vi "Read Encoder.vi"(10 "Manual Reset":bool, 11 "Encoder Ref In":T1) -> (0 "error out":errorcluster, 1 "Has Index Pulse Occured \nthis Run?":bool, 2 "Angular Encoder Abs.\nDisplacement (rad)":dbl)   [LabVIEW 2018]
uses:
  <vilib>/myRIO/Common/Instrument Driver Framework/myRIO v1.0/Encoder/typedefs/Encoder Count Direction Enum.ctl
  <vilib>/myRIO/Instrument Drivers/Onboard IO/Encoder/typedefs/Encoder Reference.ctl
  <vilib>/myRIO/Common/Instrument Driver Framework/Utilities/typedefs/myRIO Generic Hardware Reference.ctl
  <vilib>/myRIO/Common/Instrument Driver Framework/Utilities/typedefs/Hardware Version Enum.ctl
  <vilib>/myRIO/Common/Instrument Driver Framework/Utilities/typedefs/myRIO v1.0 Reference.ctl
  <vilib>/myRIO/Common/Instrument Driver Framework/Utilities/typedefs/Generic FPGA Reference.ctl
  <vilib>/myRIO/Common/Instrument Driver Framework/myRIO v1.0/Encoder/typedefs/Encoder Channels Enum.ctl
  <vilib>/Utility/error.llb/Error Cluster From Error Code.vi
  <vilib>/myRIO/Instrument Drivers/Onboard IO/Encoder/Encoder.lvlib
panel:
  out "Counter Value":i32
  out "Counter Direction":T7
  out "Angular Encoder \nDisplacement (deg)":dbl
  out "Angular Encoder Abs.\nDisplacement (deg)":dbl
  out "Overflow?":bool
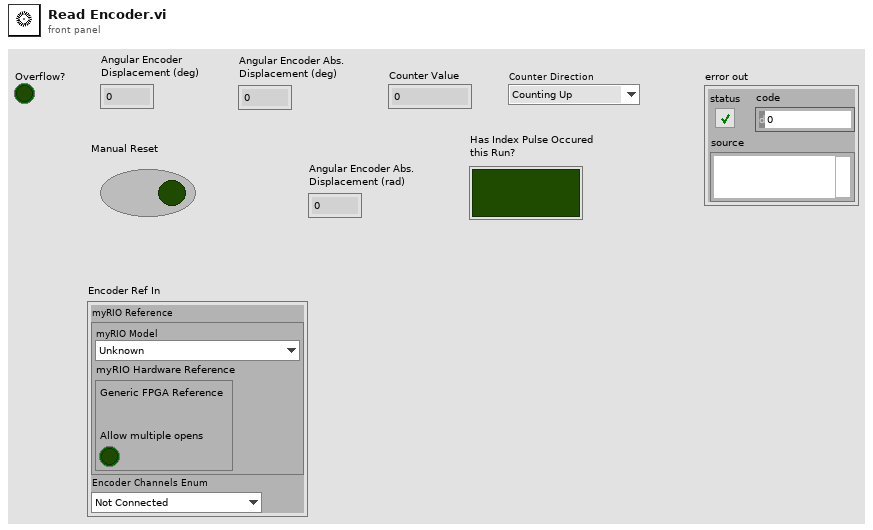
[diagram p1: front panel]
types:
  T1 = typedef "Encoder.lvlib/Encoder Reference.ctl" = cluster{"myRIO Reference":T2, "Encoder Channels Enum":T6}
  T2 = typedef "myRIO Generic Hardware Reference.ctl" = cluster{"myRIO Model":T3, "myRIO Hardware Reference":T4}
  T3 = typedef "Hardware Version Enum.ctl" = enum16{"Unknown", "myRIO-1900", "myRIO-1950", "roboRIO", "NI ELVIS RIO CM", "ELVIS III"}
  T4 = typedef "myRIO v1.0 Reference.ctl" = cluster{"Generic FPGA Reference":T5, "Allow multiple opens":bool}
  T5 = typedef "Generic FPGA Reference.ctl" = refnum<k20>
  T6 = typedef "Encoder Channels Enum.ctl" = enum16{"Not Connected", "C/ENC0", "C/ENC1", "A/ENC", "A/ENC0", "A/ENC1", "A/ENC2", "A/ENC3", "A/ENC4", "A/ENC5", "A/ENC6", "A/ENC7", "A/ENC8", "A/ENC9", "B/ENC", "B/ENC0", "B/ENC1", "B/ENC2", "B/ENC3", "B/ENC4", "B/ENC5", "B/ENC6", "B/ENC7", "B/ENC8", "B/ENC9", "DIO/ENC0", "DIO/ENC1", "DIO/ENC2", "DIO/ENC3", "DIO/ENC4"}
  T7 = typedef "Encoder Count Direction Enum.ctl" = enum16{"Counting Up", "Counting Down"}
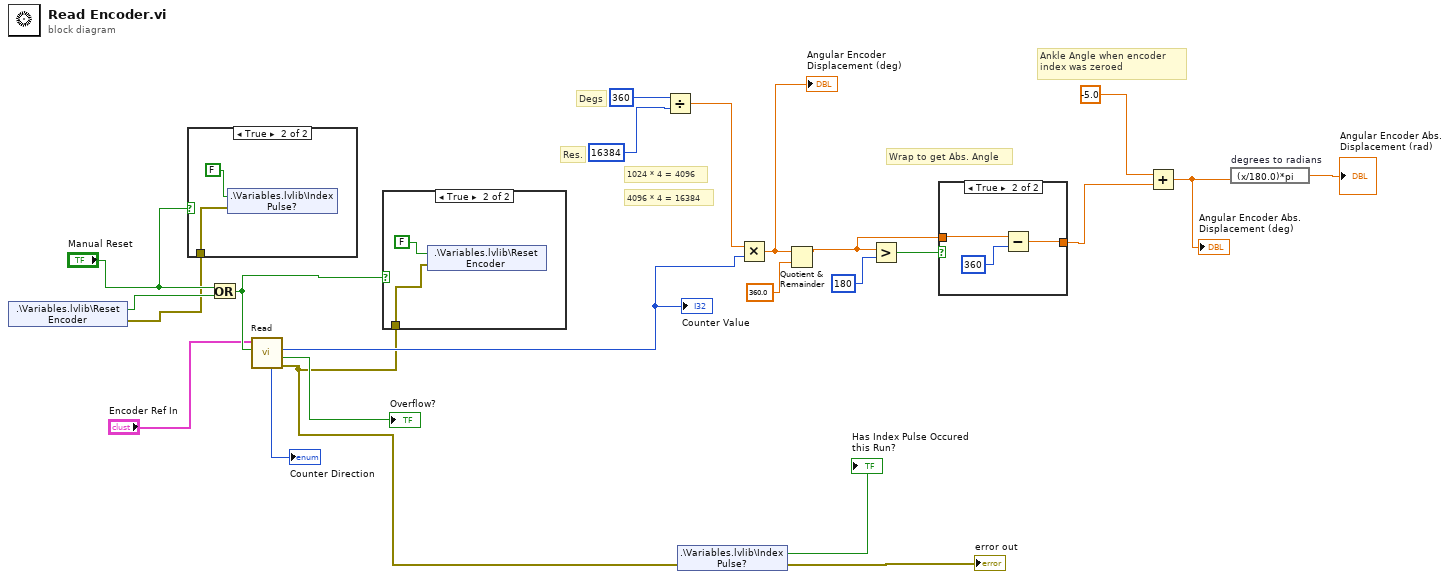
[diagram p0: block diagram]
diagram:
  # "Ankle Angle when encoder \nindex was zeroed"
  # "4096 * 4 = 16384"
  # "1024 * 4 = 4096"
  # "Wrap to get Abs. Angle"
  # "Res."
  # "Degs"
  n1 = shared-variable ".\\Variables.lvlib\\Reset Encoder"() -> (w5:bool, error out=w4:errorcluster)  [unwired: 1 in]
  n2 = case shown="True" "Manual Reset" {
    tunnel: w4 -> [_ w24]
    frame False {
    }
    frame True {
      n3 = shared-variable ".\\Variables.lvlib\\Index Pulse?"(FALSE ("Index Pulse?"), error in=w24) -> ()  [unwired: 1 out]
    }
  }
  n4 = Or(x="Manual Reset", y=w5) -> (x .or. y?=w11:bool)
  n5 = call <vilib>:"Read.vi"("Reset Counter"=w11, "Encoder Ref In"="Encoder Ref In") -> ("error out"=w9:errorcluster, "Overflow?"=→"Overflow?":bool, "Counter Value"=w14:i32, "Counter Direction"=→"Counter Direction":T7)  [unwired: 5 in, 1 out]
  "Counter Value" <- w14
  n6 = case shown="True" w11 {
    tunnel: w9 -> [_ w26]
    frame False {
    }
    frame True {
      n7 = shared-variable ".\\Variables.lvlib\\Reset Encoder"(FALSE, error in=w26) -> ()  [unwired: 1 out]
    }
  }
  n8 = Divide(x=u16 360, y=u16 16384) -> (x/y=w21:dbl)
  n9 = shared-variable ".\\Variables.lvlib\\Index Pulse?"(error in=w9) -> (→"Has Index Pulse Occured \nthis Run?":bool, error out=→"error out":errorcluster)
  n10 = Multiply(x=w21, y=w14) -> (x*y=w20:dbl)
  "Angular Encoder \nDisplacement (deg)" <- w20
  n11 = Quotient & Remainder(x=w20, y=360.0) -> (x-y*floor(x/y)=w16:dbl)  [unwired: 1 out]
  n12 = Greater?(x=w16, y=u16 180) -> (0:w17:bool)
  n13 = case shown="True" w17 {
    tunnel: w16 -> [w28 w31]
    tunnel: [w28 w29] -> w3
    frame False {
    }
    frame True {
      n14 = Subtract(x=w31, y=u16 360) -> (x-y=w29:dbl)
    }
  }
  n15 = Add(x=-5.0, y=w3) -> (x+y=w2:dbl)
  "Angular Encoder Abs.\nDisplacement (deg)" <- w2
  n16 = expression code="(x/180.0)*pi" "degrees to radians"(w2) -> (→"Angular Encoder Abs.\nDisplacement (rad)":dbl)
